vi "ERA_Main.vi"(5 "If":T1={"f_low"=0.05, "f_up"=5.0, "D_low"=0.0, "D_up"=25.0}, 7 "ERA":T2={"p_SysOdr"=2, "PMU index"=0, "dThres"=0.0}, 8 "Error In":errorcluster, 11 "Array":waveform(dbl)[](array[waveform])) -> (0 "Error Out":errorcluster, 2 "Modes":T3[](array[typedef]))   [LabVIEW 2017, in "AppPlugins.lvlib" / "EraPlugin.lvclass"]
uses:
  EraPlugin.lvclass
  Mode/Mode Content.ctl
  ERA_parameters.ctl
  COM_Select Modes Parameters.ctl
  <vilib>/Analysis/7linalg.llb/Eigenvalue and Vectors Output Option.ctl
  <vilib>/Analysis/7linalg.llb/Real Eigenvalues and Vectors.vi
  <vilib>/Analysis/NI_AALPro.lvlib
  Mode/Mode.lvclass
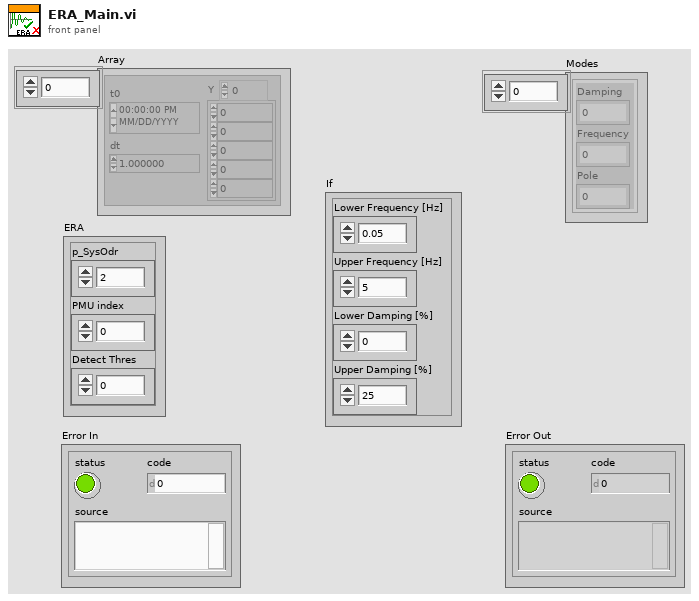
[diagram p1: front panel]
types:
  T1 = typedef "AppPlugins.lvlib/EraPlugin.lvclass/COM_Select Modes Parameters.ctl" = cluster{"f_low":dbl, "f_up":dbl, "D_low":dbl, "D_up":dbl}
  T2 = typedef "AppPlugins.lvlib/EraPlugin.lvclass/ERA_parameters.ctl" = cluster{"p_SysOdr":i32, "PMU index":i32, "dThres":dbl}
  T3 = typedef "Mode.lvclass/Mode Content.ctl" = cluster{"Damping":dbl, "Frequency":dbl, "Pole":cdb}
  T4 = typedef "NI_Matrix.lvlib/RealMatrix.ctl" = dbl[][]
  T5 = typedef "NI_AALPro.lvlib/Eigenvalue and Vectors Output Option.ctl" = i32
  T6 = cluster{"Damping":dbl, "Frequency":dbl, "Re(Pole)":dbl, "Im(Pole)":dbl}[]
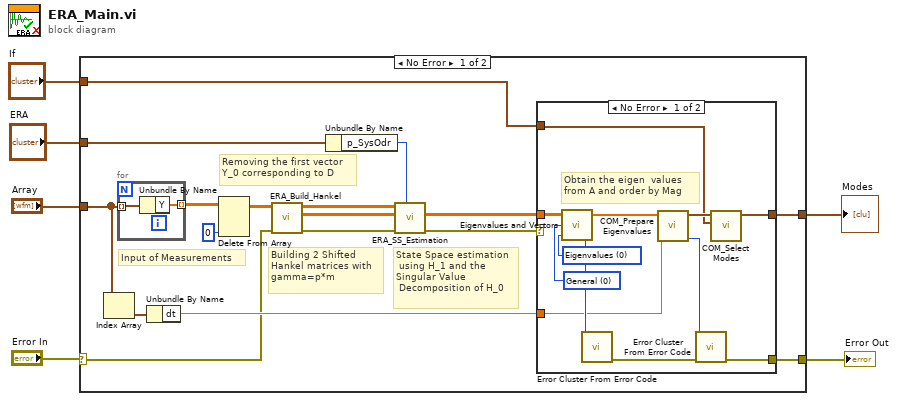
[diagram p0: block diagram]
diagram:
  n1 = case shown="No Error" "Error In" {
    selector: "Error In" -> [w8 w39]
    tunnel: "Array" -> [w16 _]
    tunnel: [w13 _] -> w5
    tunnel: "ERA" -> [w12 _]
    tunnel: [w9 w39] -> w4
    tunnel: "If" -> [w7 _]
    frame No Error {
      # "State Space estimation\n using H_1 and the \nSingular Value\n Decomposition of H_0"
      # "Building 2 Shifted \nHankel matrices with\ngamma=p*m"
      # "Removing the first vector\nY_0 corresponding to D"
      # "Input of Measurements"
      n2 = Index Array(array=w16) -> (element=w15:waveform(dbl))  [unwired: 1 in]
      n3 = for {
        tunnel: w16 -> [w38] mode=indexing
        tunnel: [w37] -> w21 mode=indexing
        n4 = Unbundle By Name(w38) -> ("Y"=w37:dbl[])
      }
      n5 = Unbundle By Name(w15) -> ("dt"=w14:dbl)
      n6 = Delete From Array(array=w21, index (col)=0 ("disabled index (col)")) -> (array with subset deleted=w22:dbl[][])  [unwired: 2 in, 1 out]
      n7 = call "ERA_Build_Hankel.vi"("error in (no error)"=w8, "Measurements"=w22) -> ("error out"=w11:errorcluster, "H_1"=w19:T4, "H_0"=w20:T4)  [unwired: 7 in]
      n8 = Unbundle By Name(w12) -> ("p_SysOdr"=w17:i32)
      n9 = call "ERA_SS_Estimation.vi"("Order Index"=w17, "Error In"=w11, "H_1"=w19, "H_0"=w20) -> ("Error Out"=w10:errorcluster, "A"=w18:T4)  [unwired: 4 in, 2 out]
      n10 = case shown="No Error" w10 {
        selector: w10 -> [_ w36]
        tunnel: w18 -> [w33 _]
        tunnel: w14 -> [w28 _]
        tunnel: [w32 _] -> w13
        tunnel: [w29 w36] -> w9
        tunnel: w7 -> [w24 _]
        frame No Error {
          w34 = T5 0 items=["Eigenvalues", "Eigenvalues & Vectors"] ("output option")
          w35 = 0 items=["General", "Symmetric"] ("matrix type")
          # "Obtain the eigen  values \nfrom A and order by Mag"
          n11 = call-poly <vilib>:"Eigenvalues and Vectors.vi"("output option"=w34, "matrix type"=w35, "Input Matrix"=w33) -> ("error"=w31:i32, "Eigenvalues"=w27:cdb[])  [unwired: 1 out]
          n12 = call <vilib>:"Error Cluster From Error Code.vi"("error code (0)"=w31) -> ("error out"=w30:errorcluster)  [unwired: 8 in]
          n13 = call "COM_Prepare Eigenvalues.vi"("dt"=w28, "Eigenvalues"=w27) -> ("error"=w25:i32, "Modes OUT"=w26:T6)  [unwired: 8 in]
          n14 = call <vilib>:"Error Cluster From Error Code.vi"("error in (no error)"=w30, "error code (0)"=w25) -> ("error out"=w29:errorcluster)  [unwired: 7 in]
          n15 = call "COM_Select Modes.vi"("Selection Parameters"=w24, "Modes IN"=w26) -> ("Modes OUT"=w32:T3[])  [unwired: 9 in]
        }
        frame Error {
        }
      }
    }
    frame Error {
    }
  }
  "Modes" <- w5
  "Error Out" <- w4
